vi "Do.vi"(8 "error in (no error)":errorcluster, 10 "Actor in":refnum<class "Actor.lvclass">, 11 "MessageRecieved Msg":refnum<class "MessageRecieved Msg.lvclass">) -> (0 "error out":errorcluster, 2 "Actor out":refnum<class "Actor.lvclass">)   [LabVIEW 2023, in "TCP_Server_Connection_Handler.lvlib" / "MessageRecieved Msg.lvclass"]
doc: "This VI delivers the message to the actor by calling the appropriate method(s) on the actor."
uses:
  MessageRecieved Msg.lvclass
  MessageRecieved Msg.lvclass/MessageRecieved Msg.ctl
  9ef47adc-f318-494c-9b8b-6df3216d6863.vi
  TCP_Connections_Controller/TCP_Connections_Controller.lvclass
  <vilib>/ActorFramework/Actor/Actor.lvclass
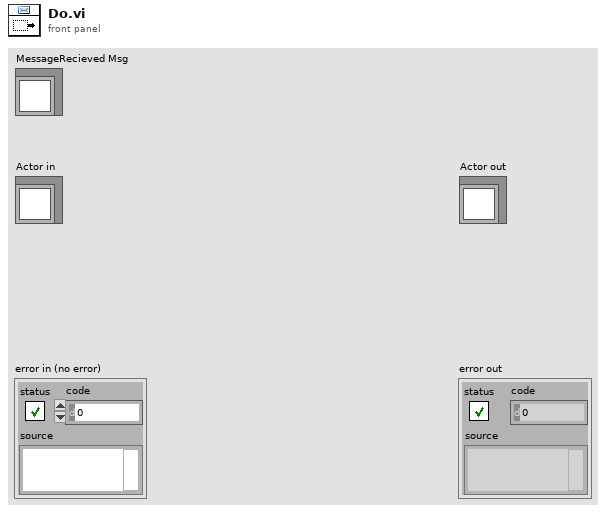
[diagram p1: front panel]
types:
  T1 = typedef "TCP_Server_Connection_Handler.lvlib/ClientMessage.ctl" = cluster{"ConnectionIndes":i32, "ClientIP":string, "Message":string}
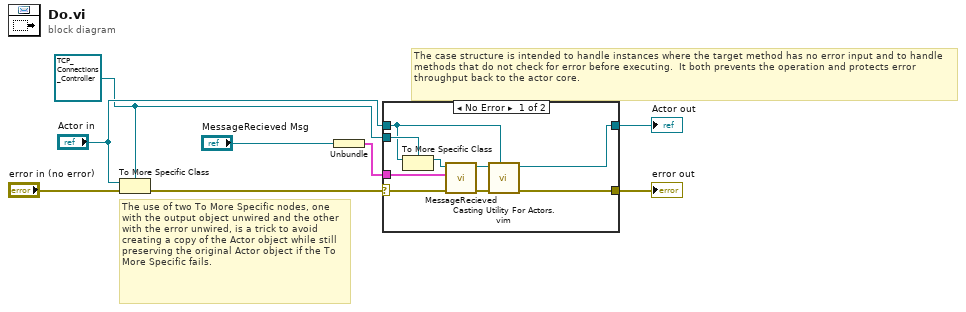
[diagram p0: block diagram]
diagram:
  w2 = refnum<class "TCP_Connections_Controller.lvclass"> refnum ("Actor in")
  # "The use of two To More Specific nodes, one with the output object unwired and the other with the error unwired, is a trick to avoid creating a copy of the Actor object while still preserving the original Actor object if the To More Specific fails."
  # "The case structure is intended to handle instances where the target method has no error input and to handle methods that do not check for error before executing.  It both prevents the operation and protects error throughput back to the actor core."
  n1 = To More Specific Class(target class=w2, reference="Actor in", error in="error in (no error)") -> (error out=w6:errorcluster)  [unwired: 1 out]
  n2 = Unbundle("MessageRecieved Msg") -> (w1:T1)
  n3 = case shown="No Error" w6 {
    selector: w6 -> [w17 w19]
    tunnel: [w11 w19] -> w5
    tunnel: [w12 w18] -> w4
    tunnel: "Actor in" -> [w14 w18]
    tunnel: w2 -> [w15 _]
    tunnel: w1 -> [w9 _]
    frame No Error {
      n4 = To More Specific Class(target class=w15, reference=w14) -> (specific class reference=w16:refnum<class "TCP_Connections_Controller.lvclass">)  [unwired: 1 in, 1 out]
      n5 = call-dynamic "MessageRecieved.vi"("error in (no error)"=w17, "clientMessage"=w9, "TCP_Connections_Controller in"=w16) -> ("error out"=w10:errorcluster, "TCP_Connections_Controller out"=w13:refnum<class "TCP_Connections_Controller.lvclass">)  [unwired: 7 in]
      n6 = call "Casting Utility For Actors.vim"("type"=w14, "error in (no error)"=w10, "Actor in"=w13) -> ("error out"=w11:errorcluster, "Actor out"=w12:refnum<class "Actor.lvclass">)  [unwired: 7 in]
    }
    frame Error {
      # "If type check fails, pass the original object out again."
    }
  }
  "error out" <- w5
  "Actor out" <- w4
